vi "HCC Panel Select Unit Type.vi"(8 "error in (no error)":errorcluster) -> (0 "error out":errorcluster, 3 "Unit Type Output":T1)   [LabVIEW 2014]
uses:
  Utility/Save File/Public/Type Definitions/Save File Unit Type.ctl
  Utility/Save File/Save File.lvlib
panel:
  in  "Complete":bool
  in  "Tab Control":enum32{"Page 1", "Page 2"}(tab)
  in  "Unit Type":T1
  # "Select Unit Type"
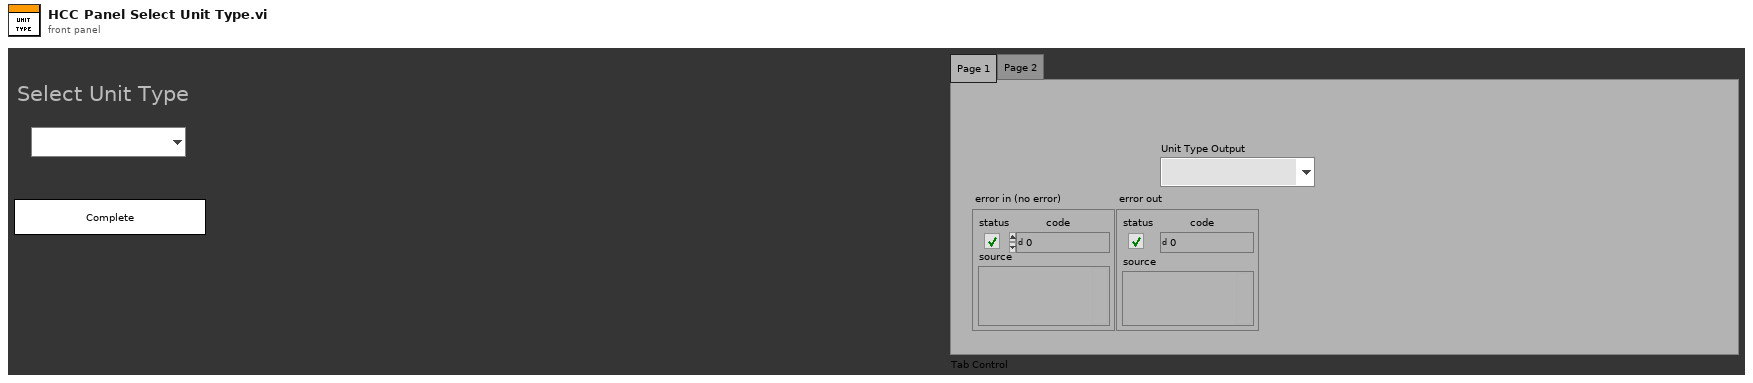
[diagram p1: front panel]
types:
  T1 = typedef "Save File.lvlib/Save File Unit Type.ctl" = enum32{"", "Viper", "Hawk", "2015", "HEWH", "Other"}
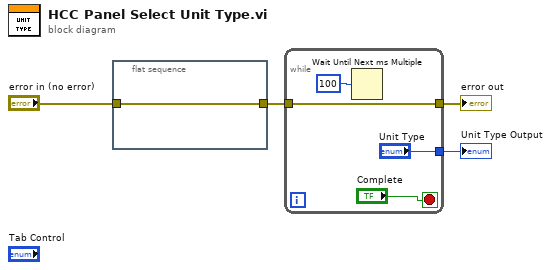
[diagram p0: block diagram]
diagram:
  n1 = flat-sequence {
    tunnel: "error in (no error)" -> [w5]
    tunnel: [w5] -> w1
    frame #0 {
    }
  }
  n2 = while {
    tunnel: ["Unit Type"] -> w4
    tunnel: w1 -> [w7]
    tunnel: [w7] -> w3
    stop <- "Complete" stop-if-true
    n3 = Wait Until Next ms Multiple(millisecond multiple=u32 100) -> ()  [unwired: 1 out]
  }
  "error out" <- w3
  "Unit Type Output" <- w4
